vi "Remove Children.vi"(8 "error in (no error)":errorcluster, 11 "Element in":refnum<class "Element.lvclass">) -> (0 "error out":errorcluster, 3 "Element out":refnum<class "Element.lvclass">)   [LabVIEW 2020, in "VILab.lvlib" / "Element.lvclass"]
uses:
  Element.lvclass
  Attribute/Attribute.lvclass
  Element.lvclass/Element.ctl
  Data Item/Data Item.lvclass
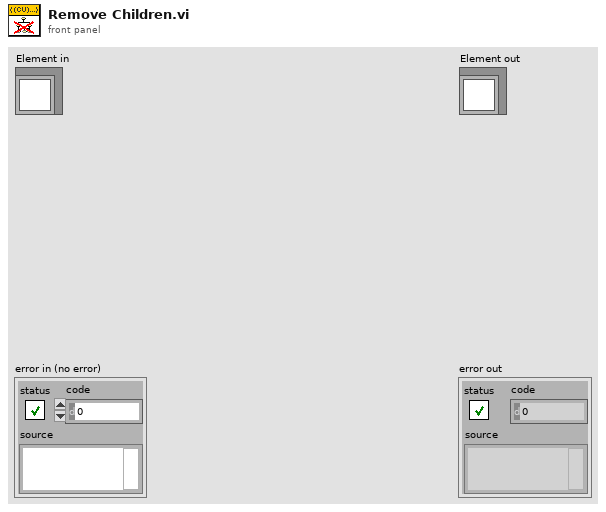
[diagram p1: front panel]
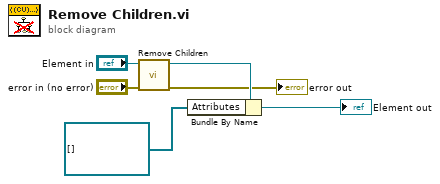
[diagram p0: block diagram]
diagram:
  n1 = call-parent "Remove Children.vi"("error in (no error)"="error in (no error)", "Data Item in"="Element in") -> ("error out"=→"error out":errorcluster, "Data Item out"=w4:refnum<class "Element.lvclass">)  [unwired: 8 in]
  n2 = Bundle By Name(cluster=w4, "Attributes"=refnum<class "Attribute.lvclass">[] []) -> (→"Element out":refnum<class "Element.lvclass">)
